vi "Calculate Bipolar Pulse Trigger.vi"(6 "pulse index":i32, 8 "error in":errorcluster, 9 "hysteresis (10%)":dbl=10.0 min=-100.0 max=100.0 step=1.0 format="%.1f", 10 "Recvy Amp (V)":dbl=-2.6339 format="%.4f", 11 "Stim Amp (V)":dbl=2.3039 format="%.4f") -> (0 "error out":errorcluster, 1 "hysteresis (V)":dbl=nan format="%.4f", 2 "trigger level (V)":dbl=nan format="%.4f", 4 "trigger slope":u16(ring)=1 items=["Falling Edge", "Rising Edge"])   [LabVIEW 2010]
panel:
  in  "edges":u16[](array[ring])=[1, 0, 0, 1] items=["Falling Edge", "Rising Edge"]
  # "Bipolar Pulse\nPattern"
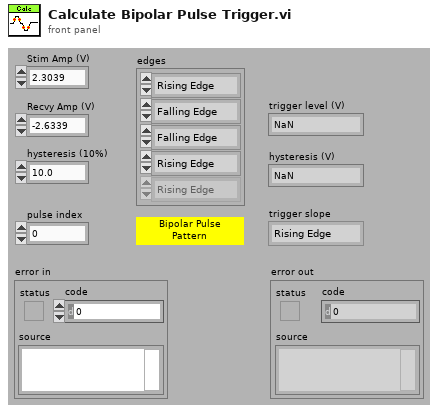
[diagram p1: front panel]
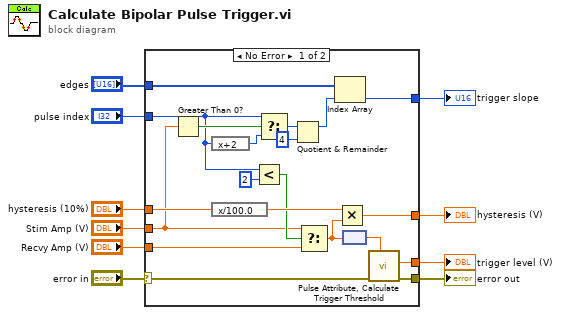
[diagram p0: block diagram]
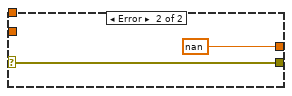
[diagram p2: hidden frame]
diagram:
  n1 = case shown="No Error" "error in" {
    selector: "error in" -> [w21 w32]
    tunnel: "edges" -> [w30 _]
    tunnel: [w29 _] -> w9
    tunnel: "pulse index" -> [w13 _]
    tunnel: "Recvy Amp (V)" -> [w15 _]
    tunnel: [w24 nan ("trigger level (V)")] -> w7
    tunnel: "Stim Amp (V)" -> [w11 _]
    tunnel: [w22 w32] -> w6
    tunnel: "hysteresis (10%)" -> [w19 _]
    tunnel: [w18 _] -> w3
    frame No Error {
      n2 = Greater Than 0?(x=w11) -> (x > 0?=w23:bool)
      n3 = expression code="x+2"(w13) -> (w28:i32)
      n4 = expression code="x/100.0"(w19) -> (w16:dbl)
      n5 = Less?(x=w13, y=2) -> (x < y?=w14:bool)
      n6 = Select(t=w13, s=w23, f=w28) -> (s? t:f=w27:i32)
      n7 = Quotient & Remainder(x=w27, y=4) -> (x-y*floor(x/y)=w25:i32)  [unwired: 1 out]
      n8 = Select(t=w11, s=w14, f=w15) -> (s? t:f=w17:dbl)
      n9 = Index Array(array=w30, index=w25) -> (element=w29:u16)
      n10 = Multiply(x=w16, y=w17) -> (x*y=w18:dbl)
      n11 = node(w17) -> (w20:dbl[unit])
      n12 = call "Pulse Attribute, Calculate Trigger Threshold.vi"("pulse amp"=w20, "error in"=w21) -> ("error out"=w22:errorcluster, "trigger level (V)"=w24:dbl)  [unwired: 5 in]
    }
    frame Error {
    }
  }
  "trigger slope" <- w9
  "trigger level (V)" <- w7
  "error out" <- w6
  "hysteresis (V)" <- w3
